vi "FTW-Test-BuildUtil-PostBuildAction.vi"() -> ()   [LabVIEW 2015]
uses:
  <vilib>/AppBuilder/AB_API_Simple/NI_App_Builder_API.lvlib
  <vilib>/AppBuilder/AB_API_Simple/Build (path).vi
panel:
  out "error out":errorcluster
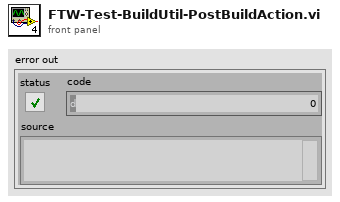
[diagram p1: front panel]
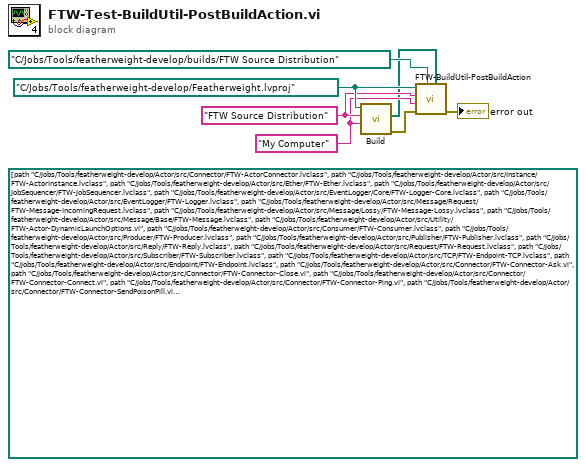
[diagram p0: block diagram]
diagram:
  w6 = path "C:/Jobs/Tools/featherweight-develop/Featherweight.lvproj" ("Project Path")
  w5 = "FTW Source Distribution" ("Build Specification Name")
  w4 = "My Computer" ("Target Name")
  (unwired) path[] [path "C:/Jobs/Tools/featherweight-develop/Actor/src/Connector/FTW-ActorConnector.lvclass", path "C:/Jobs/Tools/featherweight-develop/Actor/src/Instance/FTW-ActorInstance.lvclass", path "C:/Jobs/Tools/featherweight-develop/Actor/src/Ether/FTW-Ether.lvclass", path "C:/Jobs/Tools/featherweight-develop/Actor/src/JobSequencer/FTW-JobSequencer.lvclass", path "C:/Jobs/Tools/featherweight-develop/Actor/src/EventLogger/Core/FTW-Logger-Core.lvclass", path "C:/Jobs/Tools/featherweight-develop/Actor/src/EventLogger/FTW-Logger.lvclass", path "C:/Jobs/Tools/featherweight-develop/Actor/src/Message/Request/FTW-Message-IncomingRequest.lvclass", path "C:/Jobs/Tools/featherweight-develop/Actor/src/Message/Lossy/FTW-Message-Lossy.lvclass", path "C:/Jobs/Tools/featherweight-develop/Actor/src/Message/Base/FTW-Message.lvclass", path "C:/Jobs/Tools/featherweight-develop/Actor/src/Utility/FTW-Actor-DynamicLaunchOptions.vi", path "C:/Jobs/Tools/featherweight-develop/Actor/src/Consumer/FTW-Consumer.lvclass", path "C:/Jobs/Tools/featherweight-develop/Actor/src/Producer/FTW-Producer.lvclass", path "C:/Jobs/Tools/featherweight-develop/Actor/src/Publisher/FTW-Publisher.lvclass", path "C:/Jobs/Tools/featherweight-develop/Actor/src/Reply/FTW-Reply.lvclass", path "C:/Jobs/Tools/featherweight-develop/Actor/src/Request/FTW-Request.lvclass", path "C:/Jobs/Tools/featherweight-develop/Actor/src/Subscriber/FTW-Subscriber.lvclass", path "C:/Jobs/Tools/featherweight-develop/Actor/src/TCP/FTW-Endpoint-TCP.lvclass", path "C:/Jobs/Tools/featherweight-develop/Actor/src/Endpoint/FTW-Endpoint.lvclass", path "C:/Jobs/Tools/featherweight-develop/Actor/src/Connector/FTW-Connector-Ask.vi", path "C:/Jobs/Tools/featherweight-develop/Actor/src/Connector/FTW-Connector-Close.vi", path "C:/Jobs/Tools/featherweight-develop/Actor/src/Connector/FTW-Connector-Connect.vi", path "C:/Jobs/Tools/featherweight-develop/Actor/src/Connector/FTW-Connector-Ping.vi", path "C:/Jobs/Tools/featherweight-develop/Actor/src/Connector/FTW-Connector-SendPoisonPill.vi", path "C:/Jobs/Tools/featherweight-develop/Actor/src/Connector/FTW-Connector-SpawnNewActor.vi", path "C:/Jobs/Tools/featherweight-develop/Actor/src/Connector/FTW-Connector-Tell.vi", path "C:/Jobs/Tools/featherweight-develop/Actor/src/Instance/FTW-Actor-AddJob-Next.vi", path "C:/Jobs/Tools/featherweight-develop/Actor/src/Instance/FTW-Actor-BeginShutdownSequence.vi", path "C:/Jobs/Tools/featherweight-develop/Actor/src/Instance/FTW-Actor-Log-Event.vi", path "C:/Jobs/Tools/featherweight-develop/Actor/src/Ether/FTW-Ether-Construct.vi", path "C:/Jobs/Tools/featherweight-develop/Actor/src/Ether/FTW-Ether-CreateEphemeralPair.vi", path "C:/Jobs/Tools/featherweight-develop/Actor/src/Ether/FTW-Ether-Destroy.vi", path "C:/Jobs/Tools/featherweight-develop/Actor/src/Ether/FTW-Ether-NewLoggerConnection.vi", path "C:/Jobs/Tools/featherweight-develop/Actor/src/JobSequencer/FTW-SEQ-AddLast.vi", path "C:/Jobs/Tools/featherweight-develop/Actor/src/JobSequencer/FTW-SEQ-AddNext.vi", path "C:/Jobs/Tools/featherweight-develop/Actor/src/JobSequencer/FTW-SEQ-Construct.vi", path "C:/Jobs/Tools/featherweight-develop/Actor/src/JobSequencer/FTW-SEQ-Current.vi", path "C:/Jobs/Tools/featherweight-develop/Actor/src/JobSequencer/FTW-SEQ-Destroy.vi", path "C:/Jobs/Tools/featherweight-develop/Actor/src/JobSequencer/FTW-SEQ-GetNextStep.vi", path "C:/Jobs/Tools/featherweight-develop/Actor/src/EventLogger/Core/FTW-Logger-Process.vi", path "C:/Jobs/Tools/featherweight-develop/Actor/src/EventLogger/FTW-Logger-AddRecord.vi", path "C:/Jobs/Tools/featherweight-develop/Actor/src/EventLogger/FTW-Logger-Connect.vi", path "C:/Jobs/Tools/featherweight-develop/Actor/src/EventLogger/FTW-Logger-Launch.vi", path "C:/Jobs/Tools/featherweight-develop/Actor/src/EventLogger/FTW-Logger-Level.ctl", path "C:/Jobs/Tools/featherweight-develop/Actor/src/Message/Request/FTW-Message-Request-Body.vi", path "C:/Jobs/Tools/featherweight-develop/Actor/src/Message/Request/FTW-Message-Request-Construct.vi", path "C:/Jobs/Tools/featherweight-develop/Actor/src/Message/Request/FTW-Message-Request-Interpret.vi", path "C:/Jobs/Tools/featherweight-develop/Actor/src/Message/Request/FTW-Message-Request-Reply.vi", path "C:/Jobs/Tools/featherweight-develop/Actor/src/Message/Request/FTW-Message-Request-Unknown.vi", path "C:/Jobs/Tools/featherweight-develop/Actor/src/Message/Request/FTW-Message-Request-WriteResponse.vi", path "C:/Jobs/Tools/featherweight-develop/Actor/src/Message/Lossy/FTW-Message-Interpret.vi", path "C:/Jobs/Tools/featherweight-develop/Actor/src/Message/Lossy/FTW-Message-Lossy-CreateQueue.vi", path "C:/Jobs/Tools/featherweight-develop/Actor/src/Message/Lossy/FTW-Message-Lossy-Initialize.vi", path "C:/Jobs/Tools/featherweight-develop/Actor/src/Message/Base/FTW-Message-Initialize.vi", path "C:/Jobs/Tools/featherweight-develop/Actor/src/Message/Base/FTW-Message-Interpret.vi", path "C:/Jobs/Tools/featherweight-develop/Actor/src/Consumer/FTW-Consumer-Construct.vi", path "C:/Jobs/Tools/featherweight-develop/Actor/src/Consumer/FTW-Consumer-Destroy.vi", path "C:/Jobs/Tools/featherweight-develop/Actor/src/Producer/FTW-Producer-Construct.vi", path "C:/Jobs/Tools/featherweight-develop/Actor/src/Producer/FTW-Producer-Destroy.vi", path "C:/Jobs/Tools/featherweight-develop/Actor/src/Producer/FTW-Producer-Enqueue.vi", path "C:/Jobs/Tools/featherweight-develop/Actor/src/Publisher/FTW-Publisher-Construct.vi", path "C:/Jobs/Tools/featherweight-develop/Actor/src/Publisher/FTW-Publisher-Destroy.vi", path "C:/Jobs/Tools/featherweight-develop/Actor/src/Publisher/FTW-Publisher-Publish.vi", path "C:/Jobs/Tools/featherweight-develop/Actor/src/Reply/FTW-Reply-Construct.vi", path "C:/Jobs/Tools/featherweight-develop/Actor/src/Reply/FTW-Reply-Destroy.vi", path "C:/Jobs/Tools/featherweight-develop/Actor/src/Request/FTW-Request-Ask.vi", path "C:/Jobs/Tools/featherweight-develop/Actor/src/Request/FTW-Request-Construct.vi", path "C:/Jobs/Tools/featherweight-develop/Actor/src/Request/FTW-Request-Destroy.vi", path "C:/Jobs/Tools/featherweight-develop/Actor/src/Subscriber/FTW-Subscriber-AddAddresses.vi", path "C:/Jobs/Tools/featherweight-develop/Actor/src/Subscriber/FTW-Subscriber-Destroy.vi", path "C:/Jobs/Tools/featherweight-develop/Actor/src/Subscriber/FTW-Subscriber-Subscribe.vi", path "C:/Jobs/Tools/featherweight-develop/Actor/src/TCP/FTW-Endpoint-CreateRequester.vi", path "C:/Jobs/Tools/featherweight-develop/Actor/src/TCP/FTW-Endpoint-CreateSender.vi", path "C:/Jobs/Tools/featherweight-develop/Actor/src/TCP/FTW-Endpoint-Destroy.vi", path "C:/Jobs/Tools/featherweight-develop/Actor/src/Endpoint/FTW-Endpoint-Ask.vi", path "C:/Jobs/Tools/featherweight-develop/Actor/src/Endpoint/FTW-Endpoint-CreateReader.vi", path "C:/Jobs/Tools/featherweight-develop/Actor/src/Endpoint/FTW-Endpoint-CreateRequester.vi", path "C:/Jobs/Tools/featherweight-develop/Actor/src/Endpoint/FTW-Endpoint-CreateSender.vi", path "C:/Jobs/Tools/featherweight-develop/Actor/src/Endpoint/FTW-Endpoint-Destroy.vi", path "C:/Jobs/Tools/featherweight-develop/Actor/src/Endpoint/FTW-Endpoint-Receive.vi", path "C:/Jobs/Tools/featherweight-develop/Actor/src/Endpoint/FTW-Endpoint-Tell.vi", path "C:/Jobs/Tools/featherweight-develop/Actor/src/Connector/FTW-Connector-LaunchActor.vi", path "C:/Jobs/Tools/featherweight-develop/Actor/src/Instance/FTW-Actor-FrameworkEvent.ctl", path "C:/Jobs/Tools/featherweight-develop/Actor/src/Instance/FTW-Actor-Log-FrameworkEvent.vi", path "C:/Jobs/Tools/featherweight-develop/Actor/src/Instance/FTW-Actor-Log-Job.vi", path "C:/Jobs/Tools/featherweight-develop/Actor/src/Instance/FTW-Actor-CheckShutdown.vi", path "C:/Jobs/Tools/featherweight-develop/Actor/src/Instance/FTW-Actor-Destroy.vi", path "C:/Jobs/Tools/featherweight-develop/Actor/src/Instance/FTW-Actor-GetInstanceAddresses.vi", path "C:/Jobs/Tools/featherweight-develop/Actor/src/Instance/FTW-Actor-GetInstanceConfiguration.vi", path "C:/Jobs/Tools/featherweight-develop/Actor/src/Instance/FTW-Actor-GetNextJob.vi", path "C:/Jobs/Tools/featherweight-develop/Actor/src/Instance/FTW-Actor-HandleError.vi", path "C:/Jobs/Tools/featherweight-develop/Actor/src/Instance/FTW-Actor-Initialize.vi", path "C:/Jobs/Tools/featherweight-develop/Actor/src/Instance/FTW-Actor-Initialized.vi", path "C:/Jobs/Tools/featherweight-develop/Actor/src/Instance/FTW-Actor-LocalMessage-Worker.vi", path "C:/Jobs/Tools/featherweight-develop/Actor/src/Instance/FTW-Actor-Log-Error.vi", path "C:/Jobs/Tools/featherweight-develop/Actor/src/Instance/FTW-Actor-Publish.vi", path "C:/Jobs/Tools/featherweight-develop/Actor/src/Instance/FTW-Actor-UnknownJob.vi", path "C:/Jobs/Tools/featherweight-develop/Actor/src/Instance/FTW-Actor-LocalMessage-CheckShutdown.vi", path "C:/Jobs/Tools/featherweight-develop/Actor/src/Instance/FTW-Actor-LocalMessage-Send-Lossy.vi", path "C:/Jobs/Tools/featherweight-develop/Actor/src/Instance/FTW-Actor-LocalMessage-Send.vi", path "C:/Jobs/Tools/featherweight-develop/Actor/src/Ether/FTW-Ether-Address-Build.vi", path "C:/Jobs/Tools/featherweight-develop/Actor/src/Ether/FTW-Ether-Address-RandomEphemeral.vi", path "C:/Jobs/Tools/featherweight-develop/Actor/src/Ether/FTW-Ether-Address-Validate.vi", path "C:/Jobs/Tools/featherweight-develop/Actor/src/Ether/FTW-Ether-CreateEndpoint.vi", path "C:/Jobs/Tools/featherweight-develop/Actor/src/Ether/FTW-Ether-EndpointType.ctl", path "C:/Jobs/Tools/featherweight-develop/Actor/src/Ether/FTW-Ether-Instance.vi", path "C:/Jobs/Tools/featherweight-develop/Actor/src/Ether/FTW-Ether-MessageTransportScheme.ctl", path "C:/Jobs/Tools/featherweight-develop/Actor/src/EventLogger/Core/FTW-Logger-Construct.vi", path "C:/Jobs/Tools/featherweight-develop/Actor/src/EventLogger/Core/FTW-Logger-Destroy.vi", path "C:/Jobs/Tools/featherweight-develop/Actor/src/EventLogger/Core/FTW-Logger-FlushToFile.vi", path "C:/Jobs/Tools/featherweight-develop/Actor/src/EventLogger/Core/FTW-Logger-WriteFile.vi", path "C:/Jobs/Tools/featherweight-develop/Actor/src/EventLogger/FTW-Logger-SerializeEvent.vi", path "C:/Jobs/Tools/featherweight-develop/Actor/src/Message/Lossy/FTW-Message-Lossy-Multipart-Initialize.vi", path "C:/Jobs/Tools/featherweight-develop/Actor/src/Message/Base/FTW-Message-Compose.vi", path "C:/Jobs/Tools/featherweight-develop/Actor/src/Message/Base/FTW-Message-Decompose.vi", path "C:/Jobs/Tools/featherweight-develop/Actor/src/Message/Base/FTW-Message-Multipart-Initialize.vi", path "C:/Jobs/Tools/featherweight-develop/Actor/src/Message/Base/FTW-Message-Multipart-Interpret.vi", path "C:/Jobs/Tools/featherweight-develop/Actor/src/Consumer/FTW-Consumer-Listener.vi", path "C:/Jobs/Tools/featherweight-develop/Actor/src/Consumer/FTW-Consumer-Worker.vi", path "C:/Jobs/Tools/featherweight-develop/Actor/src/Publisher/FTW-Publisher-Listener-Start.vi", path "C:/Jobs/Tools/featherweight-develop/Actor/src/Publisher/FTW-Publisher-Listener.vi", path "C:/Jobs/Tools/featherweight-develop/Actor/src/Publisher/FTW-Publisher-Worker.vi", path "C:/Jobs/Tools/featherweight-develop/Actor/src/Reply/FTW-Reply-Listener.vi", path "C:/Jobs/Tools/featherweight-develop/Actor/src/Reply/FTW-Reply-Worker-Launch.vi", path "C:/Jobs/Tools/featherweight-develop/Actor/src/Reply/FTW-Reply-Worker.vi", path "C:/Jobs/Tools/featherweight-develop/Actor/src/Subscriber/FTW-Subscriber-Worker.vi", path "C:/Jobs/Tools/featherweight-develop/Actor/src/TCP/FTW-Endpoint-TCP-Address-Decompose.vi", path "C:/Jobs/Tools/featherweight-develop/Actor/src/TCP/FTW-Endpoint-TCP-Reply-Worker-Start.vi", path "C:/Jobs/Tools/featherweight-develop/Actor/src/TCP/FTW-Endpoint-TCP-Reply-Worker.vi", path "C:/Jobs/Tools/featherweight-develop/Actor/src/TCP/FTW-Endpoint-TCP-Request-Worker-Start.vi", path "C:/Jobs/Tools/featherweight-develop/Actor/src/TCP/FTW-Endpoint-TCP-Request-Worker.vi", path "C:/Jobs/Tools/featherweight-develop/Actor/src/TCP/FTW-Endpoint-TCP-Send-Worker-Start.vi", path "C:/Jobs/Tools/featherweight-develop/Actor/src/TCP/FTW-Endpoint-TCP-Send-Worker.vi", path "C:/Jobs/Tools/featherweight-develop/Actor/src/TCP/FTW-Endpoint-Multipart-Ask.vi", path "C:/Jobs/Tools/featherweight-develop/Actor/src/TCP/FTW-Endpoint-Multipart-Receive.vi", path "C:/Jobs/Tools/featherweight-develop/Actor/src/TCP/FTW-Endpoint-Multipart-Reply.vi", path "C:/Jobs/Tools/featherweight-develop/Actor/src/TCP/FTW-Endpoint-Multipart-Send.vi", path "C:/Jobs/Tools/featherweight-develop/Actor/src/TCP/FTW-Endpoint-Multipart-Tell.vi", path "C:/Jobs/Tools/featherweight-develop/Actor/src/TCP/FTW-Endpoint-TCP-Multipart-Ask.vi", path "C:/Jobs/Tools/featherweight-develop/Actor/src/TCP/FTW-Endpoint-Bind.vi", path "C:/Jobs/Tools/featherweight-develop/Actor/src/TCP/FTW-Endpoint-Connect.vi", path "C:/Jobs/Tools/featherweight-develop/Actor/src/TCP/FTW-Endpoint-ConnectToListener.vi", path "C:/Jobs/Tools/featherweight-develop/Actor/src/TCP/FTW-Endpoint-Listen.vi", path "C:/Jobs/Tools/featherweight-develop/Actor/src/Endpoint/FTW-Endpoint-Pipe-Construct.vi", path "C:/Jobs/Tools/featherweight-develop/Actor/src/Endpoint/FTW-Endpoint-Pipe-Flush.vi", path "C:/Jobs/Tools/featherweight-develop/Actor/src/Endpoint/FTW-Endpoint-Receive-Worker-Start.vi", path "C:/Jobs/Tools/featherweight-develop/Actor/src/Endpoint/FTW-Endpoint-Receive-Worker.vi", path "C:/Jobs/Tools/featherweight-develop/Actor/src/Endpoint/FTW-Endpoint-Multipart-Ask.vi", path "C:/Jobs/Tools/featherweight-develop/Actor/src/Endpoint/FTW-Endpoint-Multipart-Pipe-Reply.vi", path "C:/Jobs/Tools/featherweight-develop/Actor/src/Endpoint/FTW-Endpoint-Multipart-Read.vi", path "C:/Jobs/Tools/featherweight-develop/Actor/src/Endpoint/FTW-Endpoint-Multipart-Receive.vi", path "C:/Jobs/Tools/featherweight-develop/Actor/src/Endpoint/FTW-Endpoint-Multipart-Reply.vi", path "C:/Jobs/Tools/featherweight-develop/Actor/src/Endpoint/FTW-Endpoint-Multipart-Send.vi", path "C:/Jobs/Tools/featherweight-develop/Actor/src/Endpoint/FTW-Endpoint-Multipart-Tell.vi", path "C:/Jobs/Tools/featherweight-develop/Actor/src/Endpoint/FTW-Endpoint-Multipart-Write.vi", path "C:/Jobs/Tools/featherweight-develop/Actor/src/Endpoint/FTW-Endpoint-Bind.vi", path "C:/Jobs/Tools/featherweight-develop/Actor/src/Endpoint/FTW-Endpoint-Connect.vi", path "C:/Jobs/Tools/featherweight-develop/Actor/src/Endpoint/FTW-Endpoint-ConnectToListener.vi", path "C:/Jobs/Tools/featherweight-develop/Actor/src/Endpoint/FTW-Endpoint-Listen.vi", path "C:/Jobs/Tools/featherweight-develop/Core/src/Error/FTW-ERR-Clear.vi", path "C:/Jobs/Tools/featherweight-develop/Core/src/JSON/FTW-JSON-ObjectManip-AddPair.vi", path "C:/Jobs/Tools/featherweight-develop/Core/src/JSON/FTW-JSON-Construct-FromBuffer.vi", path "C:/Jobs/Tools/featherweight-develop/Core/src/JSON/FTW-JSON.lvclass", path "C:/Jobs/Tools/featherweight-develop/Core/src/JSON/FTW-JSON-UpdateMode.ctl", path "C:/Jobs/Tools/featherweight-develop/Core/src/JSON/FTW-JSON-CompareEquality.vi", path "C:/Jobs/Tools/featherweight-develop/Core/src/JSON/FTW-JSON-Core-LibraryFilepath.vi", path "C:/Jobs/Tools/featherweight-develop/Core/src/JSON/FTWLib-Jansson-Win32.dll", path "C:/Jobs/Tools/featherweight-develop/Core/src/File/FTW-File-FindLibrary.vi", path "C:/Jobs/Tools/featherweight-develop/Core/src/File/FTW-File-IsRelative.vi", path "C:/Jobs/Tools/featherweight-develop/Core/src/Error/FTW-ERR-ThrowError.vi", path "C:/Jobs/Tools/featherweight-develop/Core/src/Error/FTW-ERR-NoErrorConstant.vi", path "C:/Jobs/Tools/featherweight-develop/Core/src/Error/FTW-ERR-CallChain.vi", path "C:/Jobs/Tools/featherweight-develop/Core/src/String/FTW-STR-Array-Delimit.vi", path "C:/Jobs/Tools/featherweight-develop/Core/src/String/FTW-STR-ReplaceWhitespace.vi", path "C:/Jobs/Tools/featherweight-develop/Core/src/Regex/FTW-Regex-ReplaceAll.vi", path "C:/Jobs/Tools/featherweight-develop/Core/src/File/FTW-File-ResolveSymbolicPaths.vi", path "C:/Jobs/Tools/featherweight-develop/Core/src/Error/FTW-ERR-StatusOK.vi", path "C:/Jobs/Tools/featherweight-develop/Core/src/Regex/FTW-Regex.vi", path "C:/Jobs/Tools/featherweight-develop/Core/src/File/FTW-File-SystemDirectories.vi", path "C:/Jobs/Tools/featherweight-develop/Core/src/File/FTW-File-ValidateFilepath.vi", path "C:/Jobs/Tools/featherweight-develop/Core/src/File/FTW-File-Directory-Exists.vi", path "C:/Jobs/Tools/featherweight-develop/Core/src/File/FTW-File-ListDirectory-RegexFilter.vi", path "C:/Jobs/Tools/featherweight-develop/Core/src/File/FTW-File-ListDirectories.vi", path "C:/Jobs/Tools/featherweight-develop/Core/src/Error/FTW-ERR-StatusError.vi", path "C:/Jobs/Tools/featherweight-develop/Core/src/Regex/FTW-Regex-FilterArray.vi", path "C:/Jobs/Tools/featherweight-develop/Core/src/Error/FTW-ERR-ThrowGenericError.vi", path "C:/Jobs/Tools/featherweight-develop/Core/src/Error/FTW-ERR-ThrowImpossibleError.vi", path "C:/Jobs/Tools/featherweight-develop/Core/src/JSON/FTWLib-Jansson-Win64.dll", path "C:/Jobs/Tools/featherweight-develop/Core/src/JSON/FTWLib-Jansson-LinuxRT.so", path "C:/Jobs/Tools/featherweight-develop/Core/src/JSON/FTW-JSON-Destroy.vi", path "C:/Jobs/Tools/featherweight-develop/Core/src/JSON/FTW-JSON-Object-DeleteElement.vi", path "C:/Jobs/Tools/featherweight-develop/Core/src/JSON/FTW-JSON-Object-GetElement-Bool.vi", path "C:/Jobs/Tools/featherweight-develop/Core/src/JSON/FTW-JSON-Type.ctl", path "C:/Jobs/Tools/featherweight-develop/Core/src/JSON/FTW-JSON-Core-ElementType.vi", path "C:/Jobs/Tools/featherweight-develop/Core/src/JSON/FTW-JSON-Object-GetElement-DBL.vi", path "C:/Jobs/Tools/featherweight-develop/Core/src/JSON/FTW-JSON-Object-GetElement-Integer.vi", path "C:/Jobs/Tools/featherweight-develop/Core/src/JSON/FTW-JSON-Object-GetElement-String.vi", path "C:/Jobs/Tools/featherweight-develop/Core/src/JSON/FTW-JSON-Object-SetElement-Bool.vi", path "C:/Jobs/Tools/featherweight-develop/Core/src/JSON/FTW-JSON-Object-SetElement-DBL.vi", path "C:/Jobs/Tools/featherweight-develop/Core/src/JSON/FTW-JSON-Object-SetElement-Integer.vi", path "C:/Jobs/Tools/featherweight-develop/Core/src/JSON/FTW-JSON-Object-SetElement-String.vi", path "C:/Jobs/Tools/featherweight-develop/Core/src/JSON/FTW-JSON-Object-Update.vi", path "C:/Jobs/Tools/featherweight-develop/Core/src/JSON/FTW-JSON-Serialize.vi", path "C:/Jobs/Tools/featherweight-develop/Core/src/JSON/FTW-JSON-SetFlags-Encoding.vi", path "C:/Jobs/Tools/featherweight-develop/Core/src/JSON/FTW-JSON-Core-LibraryError.vi", path "C:/Jobs/Tools/featherweight-develop/Core/src/Reflection/FTW-Reflection-Type.vi", path "C:/Jobs/Tools/featherweight-develop/Core/src/Reflection/FTW-Reflection-Types.ctl", path "C:/Jobs/Tools/featherweight-develop/Core/src/JSON/FTW-JSON-Core-GetFlattenedValue.vi", path "C:/Jobs/Tools/featherweight-develop/Core/src/Reflection/FTW-Reflection-Cluster.vi", path "C:/Jobs/Tools/featherweight-develop/Core/src/Reflection/FTW-Reflection-Array.vi", path "C:/Jobs/Tools/featherweight-develop/Core/src/Reflection/FTW-Reflection-Enum.vi", path "C:/Jobs/Tools/featherweight-develop/Core/src/String/FTW-STR-Encode-Base64.vi", path "C:/Jobs/Tools/featherweight-develop/Core/src/JSON/FTW-JSON-Format-String.vi", path "C:/Jobs/Tools/featherweight-develop/Core/src/JSON/FTW-JSON-Escape.vi", path "C:/Jobs/Tools/featherweight-develop/Core/utils/CodeGen/JSON Deserialize/FTW-JSON-Deserialize.xnode", path "C:/Jobs/Tools/featherweight-develop/Core/utils/CodeGen/JSON Deserialize/FTW-CodeGen-State.ctl", path "C:/Jobs/Tools/featherweight-develop/Core/utils/CodeGen/JSON Deserialize/FTW-CodeGen-AdaptToInputs.vi", path "C:/Jobs/Tools/featherweight-develop/Core/utils/CodeGen/JSON Deserialize/FTW-CodeGen-Bounds.vi", path "C:/Jobs/Tools/featherweight-develop/Core/utils/CodeGen/JSON Deserialize/FTW-CodeGen-GenerateCode.vi", path "C:/Jobs/Tools/featherweight-develop/Core/utils/CodeGen/JSON Deserialize/FTW-CodeGen-Prototype.vi", path "C:/Jobs/Tools/featherweight-develop/Core/utils/CodeGen/JSON Deserialize/FTW-CodeGen-Image.vi", path "C:/Jobs/Tools/featherweight-develop/Core/utils/CodeGen/JSON Deserialize/FTW-CodeGen-Initialize.vi", path "C:/Jobs/Tools/featherweight-develop/Core/utils/CodeGen/JSON Deserialize/FTW-CodeGen-GetTerms4.vi", path "C:/Jobs/Tools/featherweight-develop/Core/utils/CodeGen/JSON Deserialize/FTW-CodeGen-UpdateStateWithRef.vi", path "C:/Jobs/Tools/featherweight-develop/Core/src/Error/FTW-ERR-StatusException.vi", path "C:/Jobs/Tools/featherweight-develop/Core/src/Error/FTW-ERR-ExceptionType.ctl", path "C:/Jobs/Tools/featherweight-develop/Core/src/Time/FTW-Time-Timer.vi", path "C:/Jobs/Tools/featherweight-develop/Core/src/Time/FTW-Time-Elapse.vi", path "C:/Jobs/Tools/featherweight-develop/Core/src/String/FTW-STR-Split.vi", path "C:/Jobs/Tools/featherweight-develop/Core/src/Time/FTW-Time-Uptime.vi", path "C:/Jobs/Tools/featherweight-develop/Core/src/Error/FTW-ERR-Ignore.vi", path "C:/Jobs/Tools/featherweight-develop/Core/src/Time/FTW-Time-DisplayFormat-Timestamp.ctl", path "C:/Jobs/Tools/featherweight-develop/Core/src/Time/FTW-Time-Display-Timestamp.vi", path "C:/Jobs/Tools/featherweight-develop/Core/src/String/FTW-STR-Random-Hex.vi", path "C:/Jobs/Tools/featherweight-develop/Core/src/File/FTW-File-CreateDirectory.vi", path "C:/Jobs/Tools/featherweight-develop/Core/src/File/FTW-File-GenerateLogFilename.vi", path "C:/Jobs/Tools/featherweight-develop/Core/src/File/FTW-File-TextWrite.vi", path "C:/Jobs/Tools/featherweight-develop/Core/src/Numeric/FTW-NUM-Counter.vi", path "C:/Jobs/Tools/featherweight-develop/Core/src/Error/FTW-ERR-SerializeForLog.vi", path "C:/Jobs/Tools/featherweight-develop/Core/src/Error/FTW-ERR-StatusCode.vi"] ("Top Level/Always Included VIs")
  n1 = call-poly <vilib>:"Build.vi"("Name of target (My Computer)"=w4, "Name of build specification (if empty: build all)"=w5, "Path to project"=w6) -> ("error out"=w3:errorcluster, "Generated files"=w1:path[])  [unwired: 7 in]
  n2 = call "FTW-BuildUtil-PostBuildAction.vi"("Files Generated by Build"=w1, "Destination Path"=path "C:/Jobs/Tools/featherweight-develop/builds/FTW Source Distribution", "error in (no error)"=w3, "Target Name"=w4, "Build Specification Name"=w5, "Project Path"=w6) -> ("error out"=→"error out":errorcluster)  [unwired: 5 in]
